vi "clock.vi"(11 "Periode µs":i16) -> ()   [LabVIEW 2019]
uses:
  <vilib>/rvi/Emulation/niFpgaGetClockAttributes.vi
  <vilib>/rvi/Emulation/niFpgaSctlEmulationGetInTimedLoop.vi
  <vilib>/rvi/Emulation/niFpgaEmulationReportErrorSimple.vi
  <vilib>/rvi/eio/common/nirviEmuTemplateMethod_errors.vi
  <vilib>/rvi/Emulation/niFpgaCriticalErrorInLSC.vi
  <vilib>/eio/EIONode/EIONode.xnode
panel:
  in  "STOP":bool
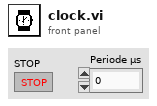
[diagram p1: front panel]
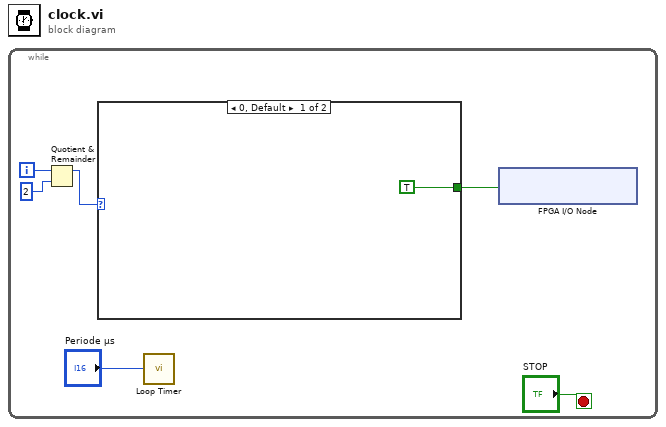
[diagram p0: block diagram]
diagram:
  n1 = while {
    i -> [w5]
    stop <- "STOP" stop-if-true
    n2 = Quotient & Remainder(x=w5, y=2) -> (x-y*floor(x/y)=w3:i32)  [unwired: 1 out]
    n3 = case shown="0, Default" w3 {
      tunnel: [TRUE _] -> w2
      frame 0, Default {
      }
      frame 1 {
      }
    }
    n4 = call "Loop Timer"("Count(uSec)"="Periode µs") -> ()  [unwired: 1 out]
    n5 = xnode "FPGA I/O Node"("ConnectorA/DIO0"=w2) -> ()  [unwired: 1 in, 1 out]
  }
